vi "GFITS_file2fitsMult.vi"(9 "def_timing":string="after", 10 "number of Extensions":u16, 11 "filename":path=path "/home/bonati/panview_current/fpas/_decam45/config/TPNT_INFO.tpl") -> (0 "number of before keys":i32[](array[numeric]), 1 "before keys":string[][][](array[string]), 2 "number of keywords":i32[](array[numeric]), 3 "Keywords":string[][][](array[string]), 4 "all keys":string[][][](array[string]), 5 "geominfo?":bool)   [LabVIEW 2016]
doc: "test"
panel:
  out "Extensions":i32[][](array[numeric])
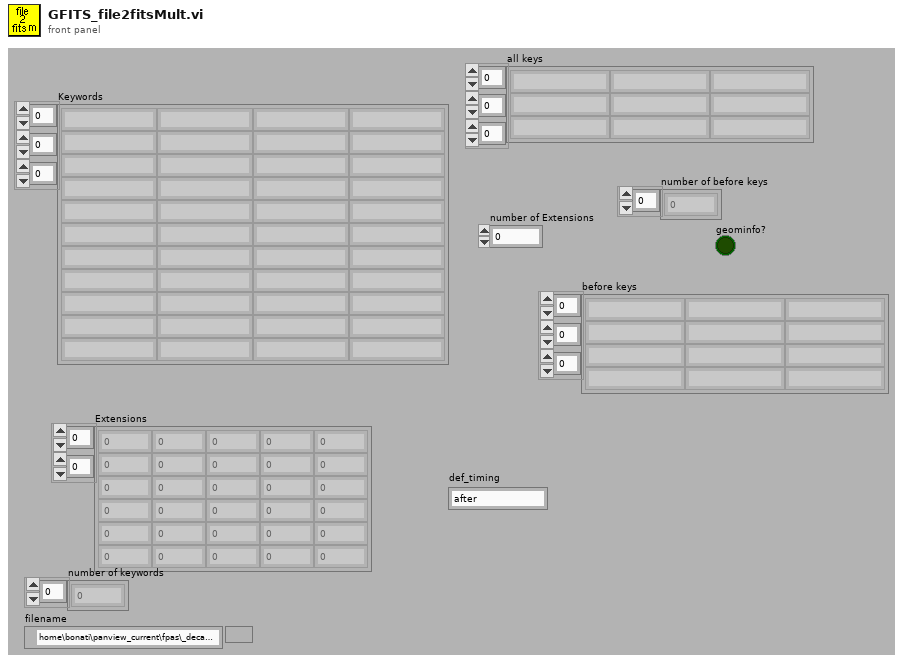
[diagram p1: front panel]
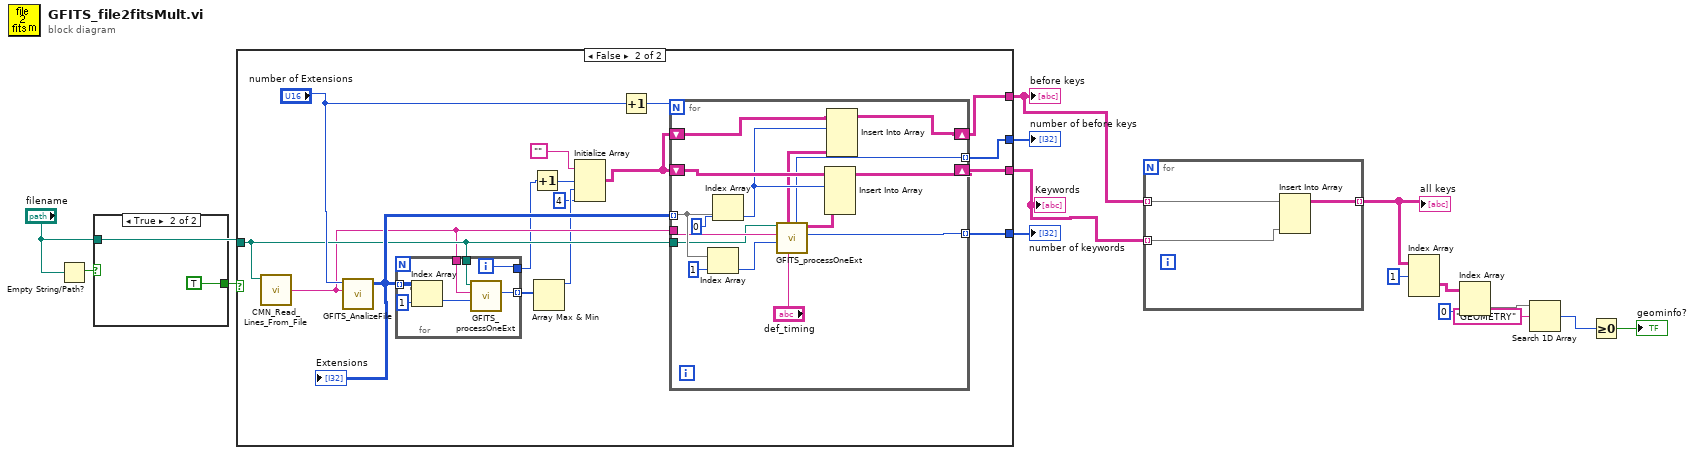
[diagram p0: block diagram]
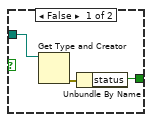
[diagram p2: hidden frame]
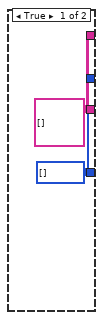
[diagram p3: hidden frame]
diagram:
  n1 = Empty String/Path?(string/path="filename") -> (empty?=w12:bool)
  n2 = case shown="True" w12 {
    tunnel: [w17 TRUE ("status")] -> w15
    tunnel: "filename" -> [w16 _]
    frame False {
      n3 = Get Type and Creator(7:w16) -> (0:w18:errorcluster)  [unwired: 1 in, 3 out]
      n4 = Unbundle By Name(w18) -> ("status"=w17:bool)
    }
    frame True {
    }
  }
  n5 = case shown="False" w15 {
    tunnel: "filename" -> [_ w30]
    tunnel: [w21 w37] -> w10
    tunnel: [w20 w36] -> w14
    tunnel: [w20 w33] -> w11
    tunnel: [w21 w32] -> w9
    frame True {
      w20 = i32[] []
      w21 = string[][][] []
      (unwired) string[][] []
      (unwired) 0
    }
    frame False {
      n6 = call "CMN_Read_Lines_From_File.vi"("file path"=w30) -> ("line string"=w29:string)  [unwired: 1 in, 7 out]
      n7 = call "GFITS_AnalizeFile.vi"("line string"=w29, "number of Extensions"="number of Extensions") -> ("Extensions"=w31:i32[][])  [unwired: 9 out]
      "Extensions" <- w31
      n8 = for {
        tunnel: w31 -> [w44] mode=indexing
        tunnel: w30 -> [w42]
        tunnel: w29 -> [w41]
        tunnel: [w39] -> w28 mode=indexing
        tunnel: [w38] -> w26
        i -> [w38]
        n9 = Index Array(array=w44, index=1) -> (element=w40:i32)
        n10 = call "GFITS_processOneExt.vi"("starting line"=w40, "line string"=w41, "config file"=w42) -> ("number of keywords"=w39:i32)  [unwired: 1 in, 7 out]
      }
      n11 = Increment(x=w26) -> (x+1=w25:i32)
      n12 = Array Max & Min(array=w28) -> (max value=w27:i32)  [unwired: 3 out]
      n13 = Initialize Array("", w25, w27, 4 ("dimension size")) -> (w23:string[][][])
      n14 = Increment(x="number of Extensions") -> (x+1=w35:u16)
      n15 = for {
        N: w35 -> [_]
        shift-right: [w52] -> w37
        shift-left: w23 -> [w55]
        tunnel: w31 -> [w60] mode=indexing
        tunnel: w29 -> [w57]
        tunnel: [w53] -> w36 mode=indexing
        shift-right: [w46] -> w32
        shift-left: w23 -> [w47]
        tunnel: [w48] -> w33 mode=indexing
        tunnel: w30 -> [w45]
        n16 = Index Array(array=w60, index=1 ("Index")) -> (element=w56:i32)
        n17 = Index Array(array=w60, index=0 ("Index")) -> (element=w50:i32)
        n18 = call "GFITS_processOneExt.vi"("def_timing"="def_timing", "starting line"=w56, "line string"=w57, "config file"=w45) -> ("number of keywords"=w53:i32, "Extension Keywords"=w54:string[][], "number of before keywords"=w48:i32, "Extension before keywords"=w49:string[][])  [unwired: 4 out]
        n19 = Insert Into Array(array=w55, index (dim 0)=w50, new element=w54) -> (w52:string[][][])  [unwired: 2 in]
        n20 = Insert Into Array(array=w47, index (dim 0)=w50, new element=w49) -> (w46:string[][][])  [unwired: 2 in]
      }
    }
  }
  "Keywords" <- w10
  "number of keywords" <- w14
  "number of before keys" <- w11
  "before keys" <- w9
  n21 = for {
    tunnel: w10 -> [w63] mode=indexing
    tunnel: w9 -> [w62] mode=indexing
    tunnel: [w61] -> w8 mode=indexing
    n22 = Insert Into Array(array=w62, new element=w63) -> (w61:string[][])  [unwired: 2 in]
  }
  "all keys" <- w8
  n23 = Index Array(array=w8, index (dim 0)=1 ("index (page)")) -> (element=w1:string[][])  [unwired: 2 in]
  n24 = Index Array(array=w1, index (col)=0 ("disabled index (col)")) -> (element=w5:string[])  [unwired: 1 in]
  n25 = Search 1D Array(1D array=w5, element="GEOMETRY") -> (index of element=w3:i32)  [unwired: 1 out]
  n26 = Greater Or Equal To 0?(x=w3) -> (x >= 0?=→"geominfo?":bool)
